vi "Device Information.vi"(8 "error in (no error)":errorcluster, 10 "id":string, 11 "particle reference in":T1) -> (0 "error out":errorcluster, 2 "device query JSON":T3, 3 "particle reference out":T1)   [LabVIEW 2013, in "Particle API.lvlib"]
doc: "Query the currently connected Spark device for basic information."
uses:
  Particle API.lvlib
  Controls/Device Query JSON.ctl
  Controls/Particle Reference.ctl
  <vilib>/httpClient/ClientHandle.ctl
  <vilib>/httpClient/LabVIEWHTTPClient.lvlib
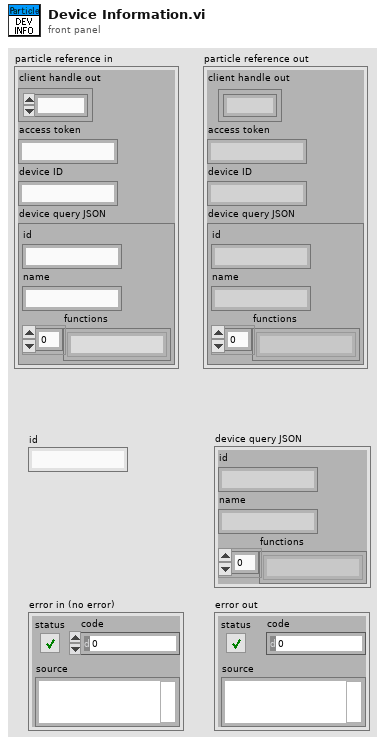
[diagram p1: front panel]
types:
  T1 = typedef "Particle API.lvlib/Particle Reference.ctl" = cluster{"client handle out":T2, "access token":string, "device ID":string, "device query JSON":T3}
  T2 = typedef "LabVIEWHTTPClient.lvlib/ClientHandle.ctl" = refnum<k1>
  T3 = typedef "Particle API.lvlib/Device Query JSON.ctl" = cluster{"id":string, "name":string, "functions":string[]}
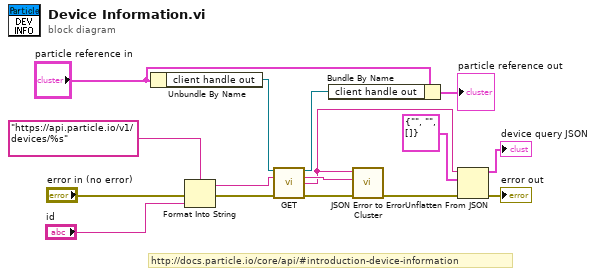
[diagram p0: block diagram]
diagram:
  # "http://docs.particle.io/core/api/#introduction-device-information"
  n1 = Unbundle By Name("particle reference in") -> ("client handle out"=w2:T2)
  n2 = Format Into String(format string="https://api.particle.io/v1/devices/%s" ("url"), error in="error in (no error)", "id") -> (resulting string=w6:string, error out=w5:errorcluster)  [unwired: 1 in]
  n3 = call <vilib>:"GET.vi"("client handle"=w2, "url"=w6, "error in (no error)"=w5) -> ("client handle out"=w1:T2, "headers"=w16:string, "body"=w15:string, "error out"=w13:errorcluster)  [unwired: 9 in]
  n4 = Bundle By Name(cluster="particle reference in", "client handle out"=w1) -> (→"particle reference out":T1)
  n5 = call "JSON Error to Error Cluster.vi"("error in (no error)"=w13, "headers"=w16, "JSON string"=w15) -> ("error out"=w14:errorcluster)  [unwired: 8 in]
  n6 = Unflatten From JSON(JSON string=w15, type and defaults=T3 {"id"="", "name"="", "functions"=[]} ("Device Query JSON"), error in (no error)=w14) -> (value=→"device query JSON":T3, error out=→"error out":errorcluster)  [unwired: 4 in]
